vi "LIA PLL Simulation Raw Data.vi"() -> ()   [LabVIEW 2017]
uses:
  <instrlib>/_niInstr/Data Trigger/v1/Shared/Public/Edge Configuration FXP(+-,18,1).ctl
  <instrlib>/_niInstr/Data Trigger/v1/Shared/Public/Edge Configuration Trigger Slope.ctl
  <instrlib>/_niInstr/Data Trigger/v1/Shared/niInstr Data Trigger v1 Shared.lvlib
panel:
  out "q":dbl
  in  "signal freq":dbl=100000.0 format="%#_6p"
  out "# samples":dbl format="%#_f"
  in  "Tab Control":enum32{"PLL", "Lock-In Signal", "CIC"}(tab)
  out "Accumulator":dbl format="%_12f"
  out "Frequency (f/Fs)":dbl format="%_12f"
  out "Frequency (f/Fs) Graph":dbl(graph)
  in  "Delay Time (s)":dbl=0.0001 format="%#_13g"
  out "PLL Source":dbl(graph)
  out "progress":dbl(slide) scale=0.0..1.0
  in  "stop":bool
  in  "pll.arm":bool
  in  "pll.m":i8=-20
  in  "pll.config":T1={"highLevel"=0.25, "lowLevel"=0.0, "trigger slope"=enum."Positive"}
  in  "pll.reset":bool
  in  "file path":path=path "C:/Repositories/Lock-In-Amplifier/tmds/raw-adc-data-00.tdms"
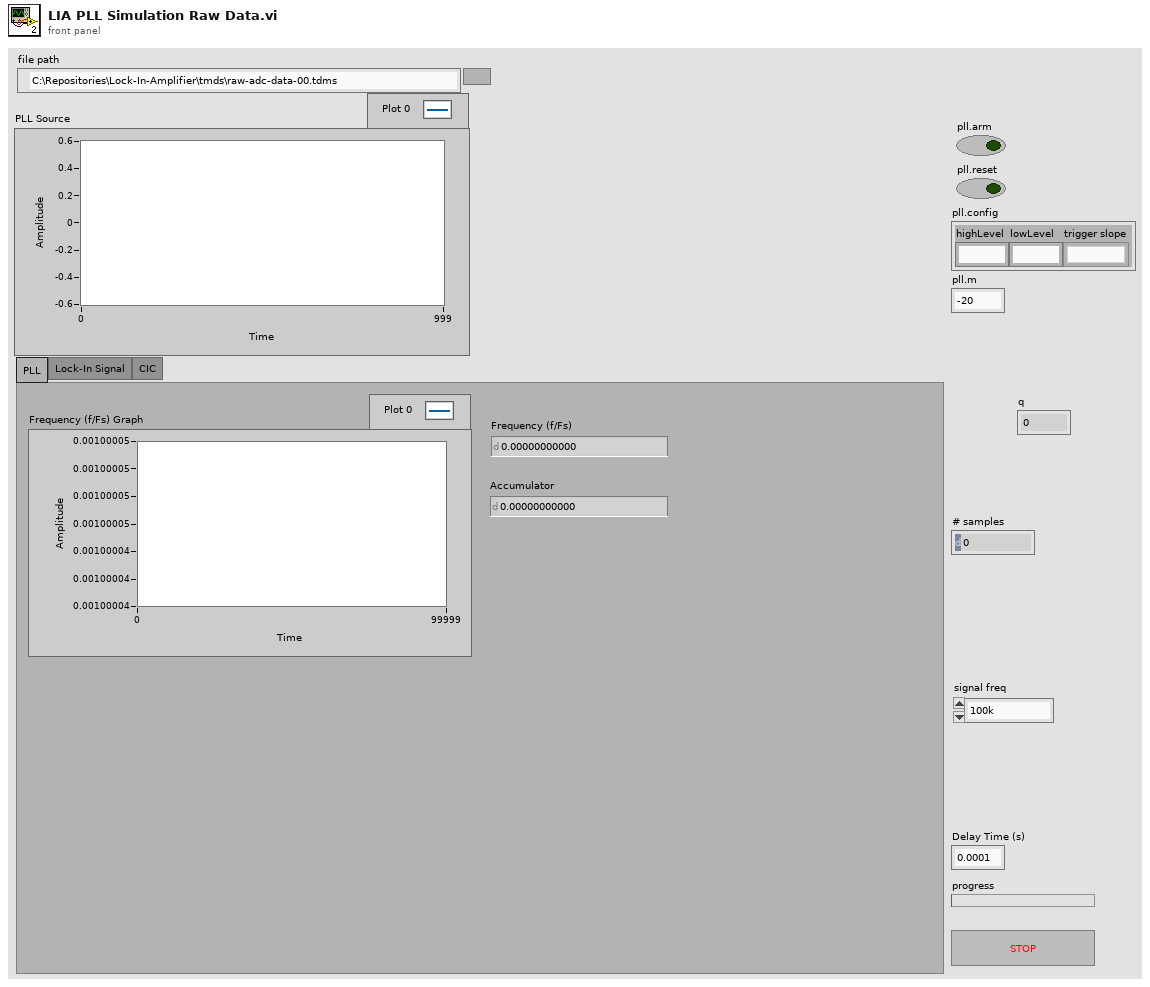
[diagram p1: front panel]
types:
  T1 = typedef "niInstr Data Trigger v1 Shared.lvlib/Edge Configuration FXP(+-,18,1).ctl" = cluster{"highLevel":fxp<+/-,18,1>, "lowLevel":fxp<+/-,18,1>, "trigger slope":T2}
  T2 = typedef "niInstr Data Trigger v1 Shared.lvlib/Edge Configuration Trigger Slope.ctl" = enum8{"Positive", "Negative"}
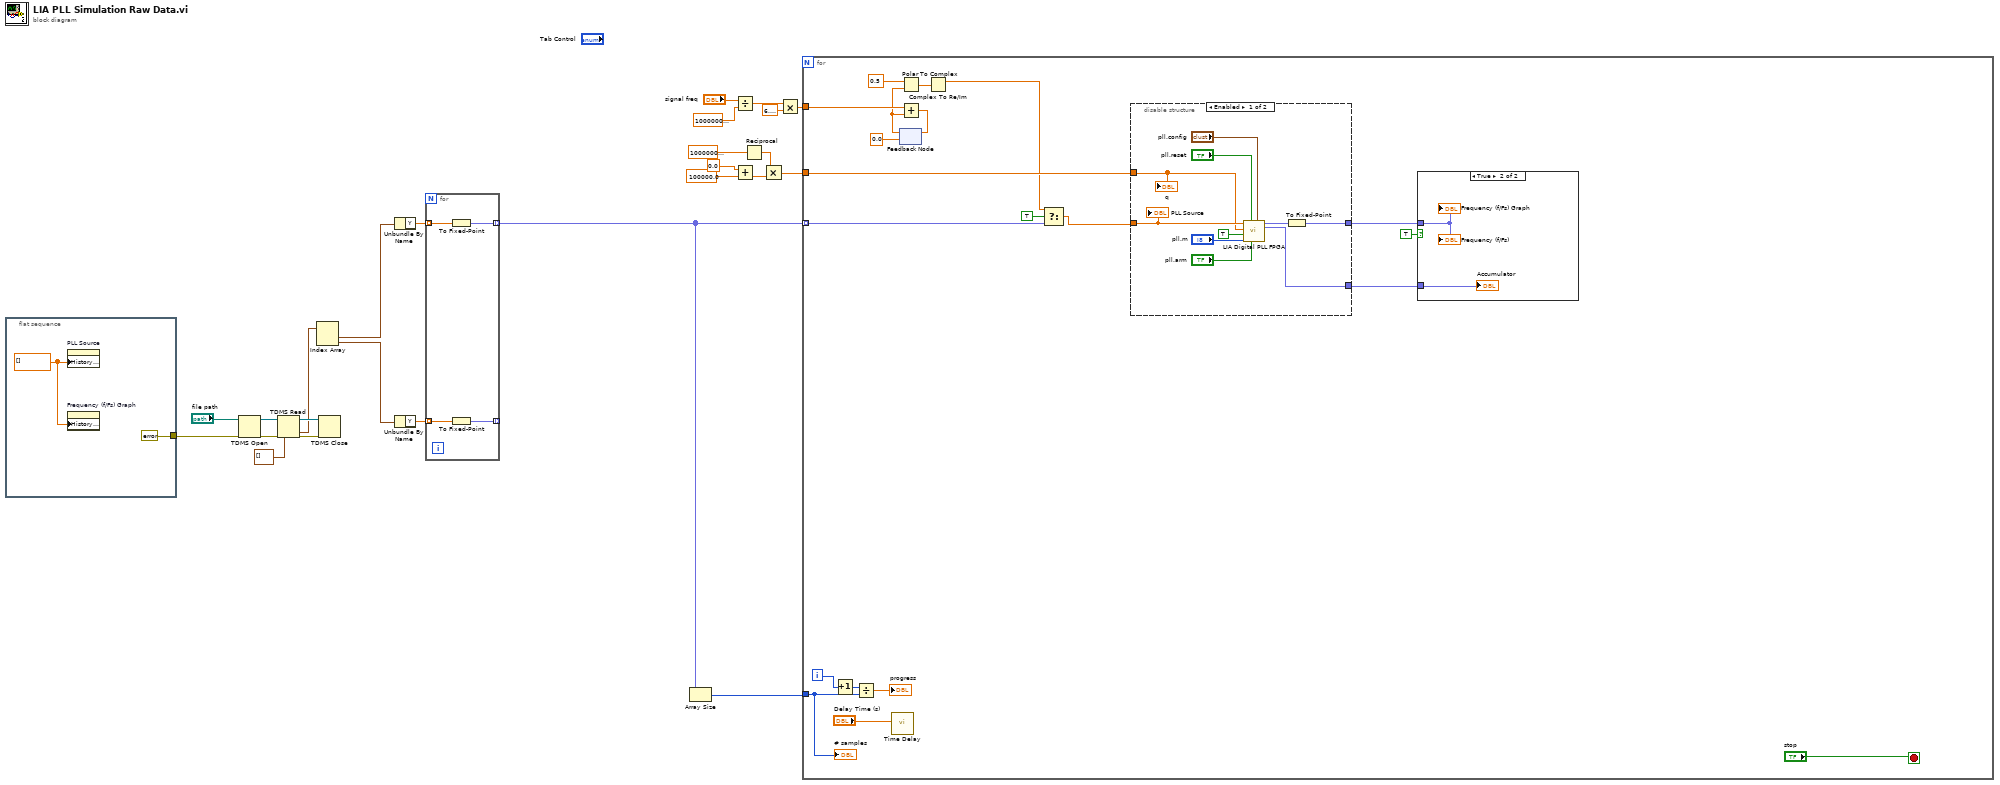
[diagram p0: block diagram]
diagram:
  n1 = flat-sequence {
    tunnel: [errorcluster {"status"=FALSE, "code"=0, "source"=""} ("error constant")] -> w13
    frame #0 {
      w26 = dbl[] [] ("History Data")
      n2 = property on="PLL Source" class="WFChart (strict)"("History Data"=w26) -> ()  [unwired: 2 in, 2 out]
      n3 = property on="Frequency (f/Fs) Graph" class="WFChart (strict)"("History Data"=w26) -> ()  [unwired: 2 in, 2 out]
    }
  }
  n4 = TDMS Open(8:w13, 11:"file path") -> (0:w23:errorcluster, 3:w24:refnum<k34>)  [unwired: 5 in]
  n5 = TDMS Read(0:w24, 11:w23, 12:waveform(dbl)[] []) -> (4:w21:refnum<k34>, 10:w19:waveform(dbl)[], 15:w20:errorcluster)  [unwired: 5 in, 3 out]
  n6 = Index Array(array=w19) -> (element #1=w18:waveform(dbl), element #2=w15:waveform(dbl))  [unwired: 2 in]
  n7 = TDMS Close(8:w20, 11:w21) -> ()  [unwired: 2 out]
  n8 = Unbundle By Name(w18) -> ("Y"=w17:dbl[])
  n9 = Unbundle By Name(w15) -> ("Y"=w16:dbl[])
  n10 = for {
    tunnel: w17 -> [w31] mode=indexing
    tunnel: [w30] -> w1 mode=indexing
    tunnel: w16 -> [w29] mode=indexing
    tunnel: [w28] -> _ mode=indexing
    n11 = To Fixed-Point(number=w31) -> (fixed-point=w30:fxp<+/-,18,1>)  [unwired: 1 in]
    n12 = To Fixed-Point(number=w29) -> (fixed-point=w28:fxp<+/-,18,1>)  [unwired: 1 in]
  }
  n13 = Array Size(array=w1) -> (size(s)=w14:i32)
  n14 = Divide(x="signal freq", y=100000000.0 ("x")) -> (x/y=w7:dbl)
  n15 = Add(x=0.0, y=100000.0) -> (x+y=w3:dbl)
  n16 = Reciprocal(x=100000000.0) -> (1/x=w11:dbl)
  n17 = Multiply(x=w11, y=w3) -> (x*y=w9:dbl)
  n18 = Multiply(x=w7, y=6.283185307179586) -> (x*y=w4:dbl)
  n19 = for {
    tunnel: w1 -> [w34] mode=indexing
    tunnel: w14 -> [w46]
    tunnel: w9 -> [w47]
    tunnel: w4 -> [w42]
    i -> [w45]
    stop <- "stop" stop-if-true
    n20 = Increment(x=w45) -> (x+1=w50:i32)
    n21 = Divide(x=w50, y=w46) -> (x/y=→"progress":dbl)
    n22 = call "Time Delay"("Delay Time (s)"="Delay Time (s)") -> ()  [unwired: 10 in, 1 out]
    n23 = feedback #1(0.0 ("r")) -> (w37:dbl)
    n24 = Polar To Complex(1:w37, 2:0.5 ("r")) -> (0:w36:cdb)
    n25 = Add(x=w42, y=w37) -> (x+y=w38:dbl)
    n26 = feedback-in #1(w38) -> ()
    n27 = Complex To Re/Im(x + iy=w36) -> (x=w32:dbl)  [unwired: 1 out]
    n28 = Select(t=w32, s=TRUE, f=w34) -> (s? t:f=w33:dbl)
    n29 = disable-structure shown="Enabled" {
      disable-tunnel: w33 -> [w58 _]
      disable-tunnel: [w56 w64] -> w43
      disable-tunnel: w47 -> [w57 w64]
      disable-tunnel: [w54 _] -> w41
      frame Enabled {
        n30 = call "LIA Digital PLL FPGA.vi"("configuration"="pll.config", "arm"="pll.arm", "reset"="pll.reset", "m"="pll.m", "input valid"=TRUE, "q"=w57, "I"=w58) -> ("accumulator"=w54:fxp<+/-,48,0>, "frequency shift"=w55:fxp<+/-,48,0>)  [unwired: 1 in, 2 out]
        n31 = To Fixed-Point(number=w55) -> (fixed-point=w56:fxp<+/-,48,0>)  [unwired: 1 in]
        "PLL Source" <- w58
        "q" <- w57
      }
      frame Disabled {
      }
    }
    n32 = case shown="True" TRUE {
      tunnel: w43 -> [_ w53]
      tunnel: w41 -> [_ w52]
      frame False {
      }
      frame True {
        "Frequency (f/Fs) Graph" <- w53
        "Frequency (f/Fs)" <- w53
        "Accumulator" <- w52
      }
    }
    "# samples" <- w46
  }
